vi "Main.vi"() -> ()   [LabVIEW 2022 SP3]
uses:
  Estados.ctl
panel:
  in  "Stop Button":bool
  in  "Tab Control":enum32{"Test Sequence", "SysConfig"}(tab)
  out "TestSeq":string[][](table)
  in  "StopOnFail":bool caption="Stop on fail"
  in  "SNLen":i32 caption="Barcode Lenght"
  in  "ScanComPort":i32 caption="Scanner Com port"
  in  "Enable Trac":bool caption="Traceability Enable"
  in  "Save":bool
  in  "SysPwd":string caption="Password"
  in  "Station":string caption="Station Name"
  out "Cimplicity":bool caption="Cimplicity Status"
  out "image":picture
  out "OperMsg":string caption="Operator Message"
  in  "Serial":string caption="Barcode SN"
  # "IPB2 Test Sequencer"
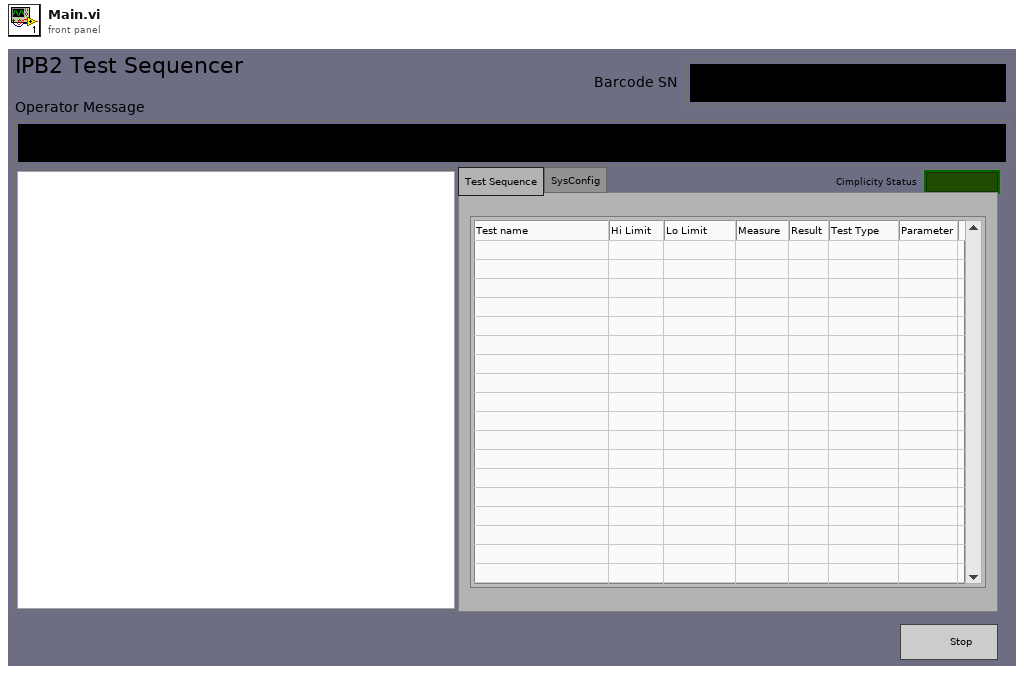
[diagram p1: front panel]
types:
  T1 = typedef "Estados.ctl" = enum16{"Standby", "ScanLabel", "Backcheck", "CloseFixture", "PerfomTest", "SendResult", "End"}
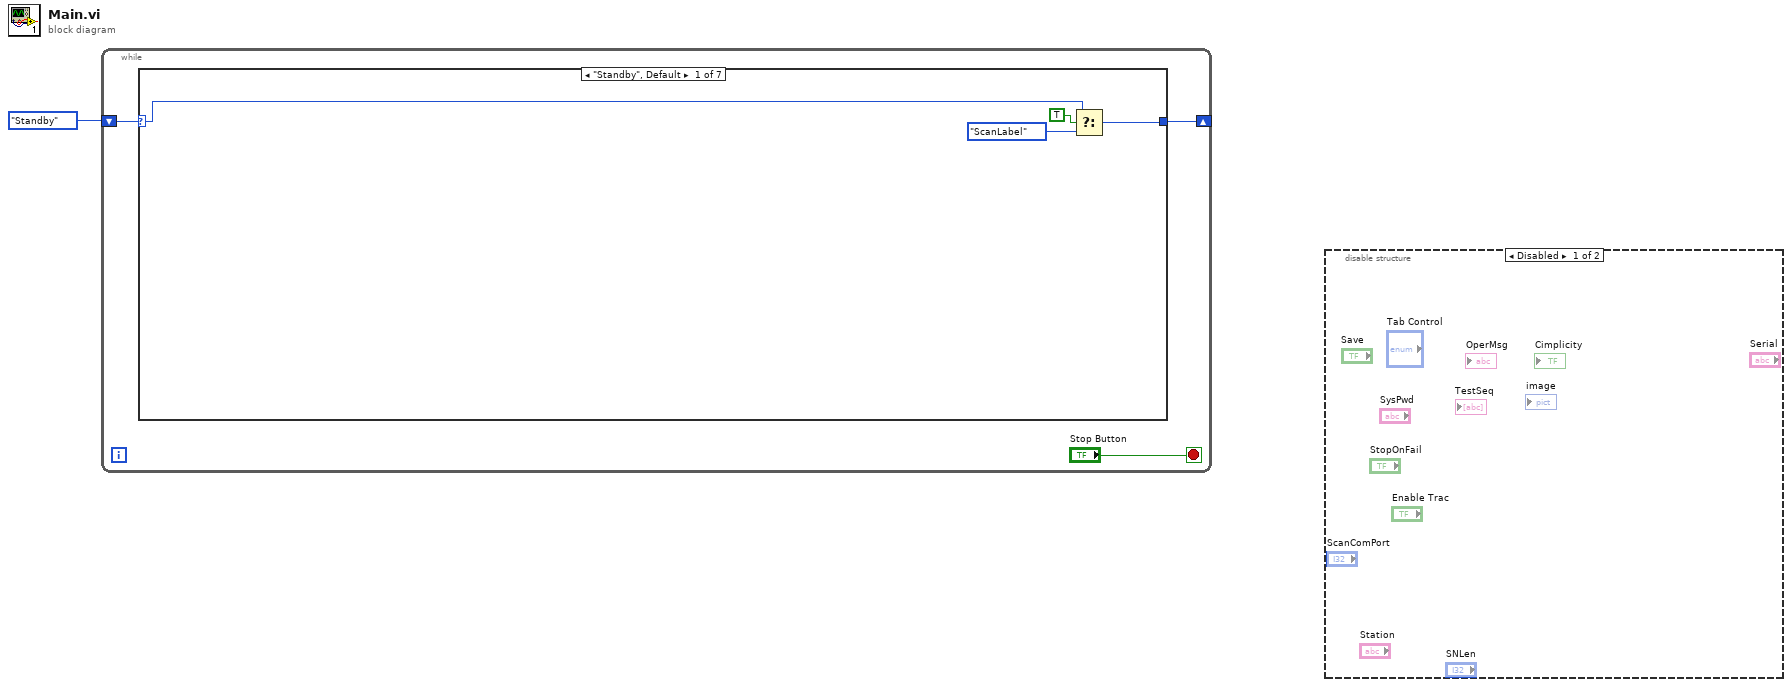
[diagram p0: block diagram]
diagram:
  n1 = while {
    shift-right: [w2] -> _
    shift-left: Estados."Standby" -> [w3]
    stop <- "Stop Button" stop-if-true
    n2 = case shown="\"Standby\", Default" w3 {
      selector: w3 -> [w6 _ _ _ _ _ _]
      tunnel: [w8 _ _ _ _ _ _] -> w2
      frame "Standby", Default {
        n3 = Select(t=w6, s=TRUE, f=Estados."ScanLabel") -> (s? t:f=w8:T1)
      }
      frame "ScanLabel" {
      }
      frame "Backcheck" {
      }
      frame "CloseFixture" {
      }
      frame "PerfomTest" {
      }
      frame "SendResult" {
      }
      frame "End" {
      }
    }
  }
  n4 = disable-structure shown="Disabled" {
    frame Disabled {
    }
    frame Enabled {
    }
  }
